vi "Base_Method1.vi"(8 "error in (no error)":errorcluster, 11 "Base1 in":refnum<class "Base1.lvclass">) -> (0 "error out":errorcluster, 3 "Base1 out":refnum<class "Base1.lvclass">)   [LabVIEW 2020, in "RootLibrary.lvlib" / "Base1Library.lvlib" / "Base1.lvclass"]
uses:
  Base1.lvclass
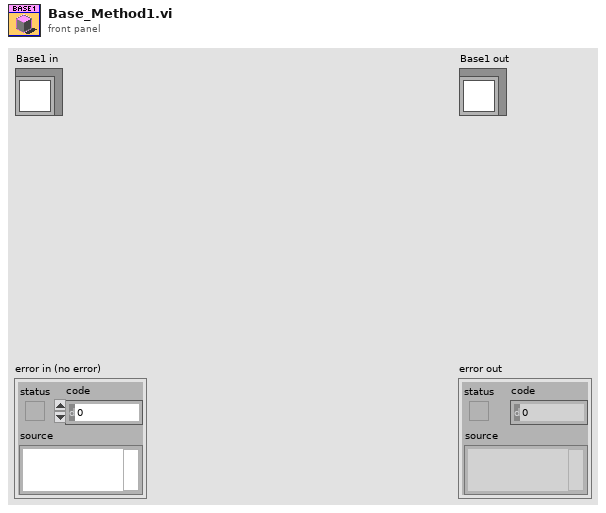
[diagram p1: front panel]
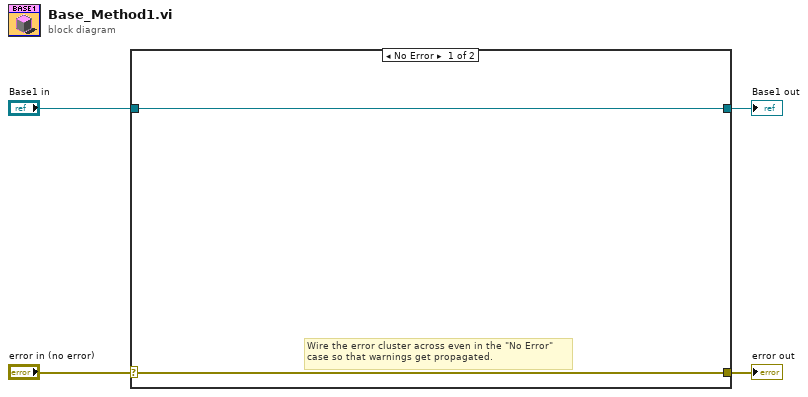
[diagram p0: block diagram]
diagram:
  n1 = case shown="No Error" "error in (no error)" {
    selector: "error in (no error)" -> [w5 w8]
    tunnel: [w5 w8] -> w3
    tunnel: [w6 w7] -> w1
    tunnel: "Base1 in" -> [w6 w7]
    frame No Error {
      # "Wire the error cluster across even in the \"No Error\"\ncase so that warnings get propagated."
    }
    frame Error {
    }
  }
  "error out" <- w3
  "Base1 out" <- w1
